vi "nc_get_NC.vi"(3 "ErrorIn":errorcluster caption="Error in", 5 "FilePath":path) -> (0 "ErrorOut":errorcluster caption="error out", 1 "NC":T1 {"vars"."NC_attrarray"."nc_type" items=["NC_NAT", "NC_BYTE", "NC_CHAR", "NC_SHORT", "NC_INT", "NC_FLOAT", "NC_DOUBLE"]; "attrs"."nc_type" items=["NC_NAT", "NC_BYTE", "NC_CHAR", "NC_SHORT", "NC_INT", "NC_FLOAT", "NC_DOUBLE"]}, 2 "refnum out":refnum<file>)   [LabVIEW 2016]
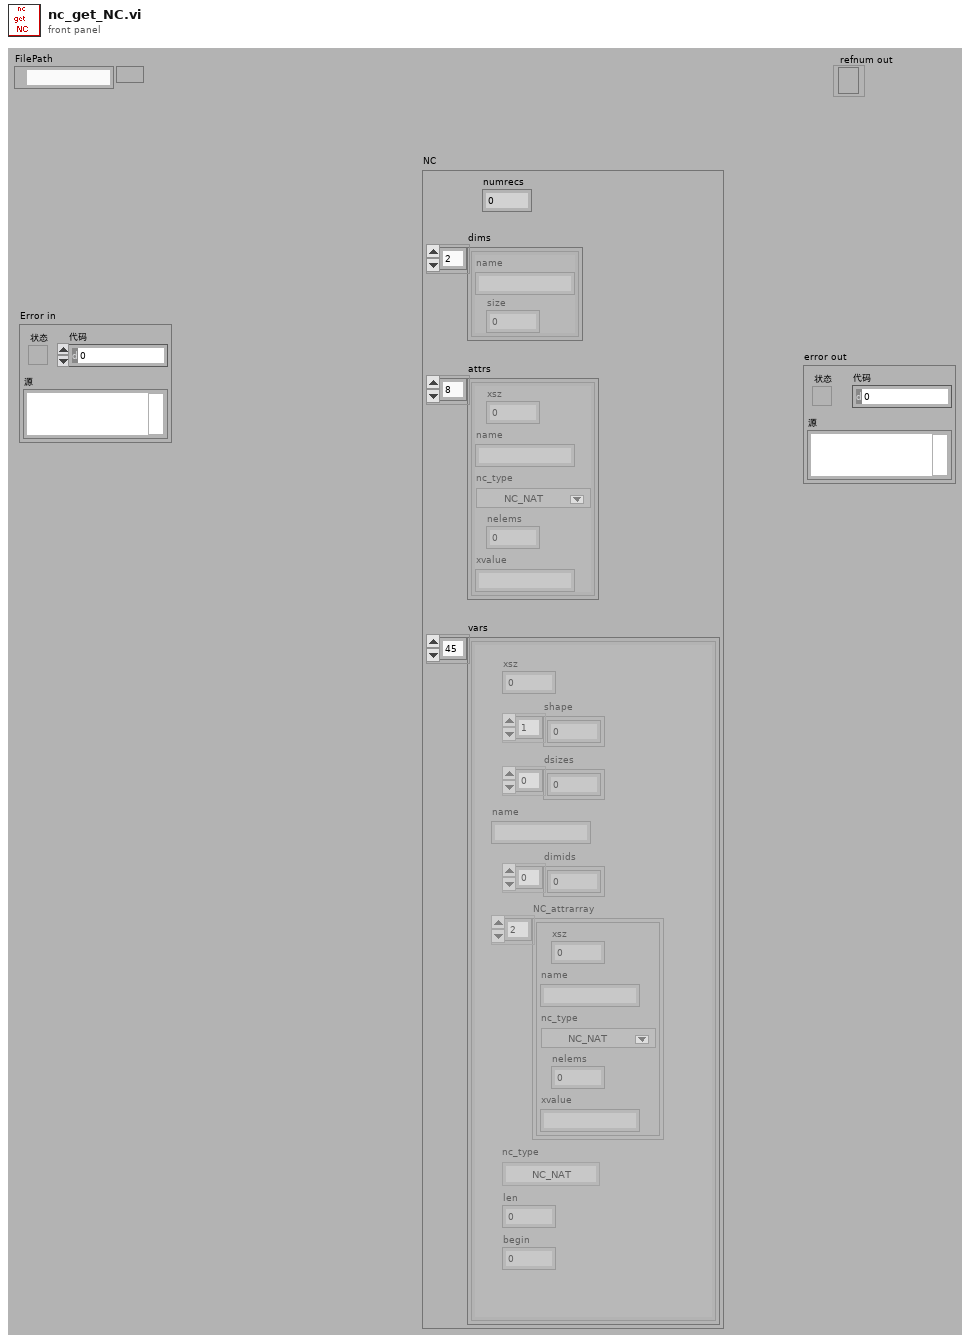
[diagram p1: front panel]
types:
  T1 = cluster{"numrecs":u64, "dims":cluster{"name":string, "size":u64}[], "attrs":cluster{"xsz":u64, "name":string, "nc_type":u16, "nelems":u64, "xvalue":string}[], "vars":cluster{"xsz":u64, "shape":u64[], "dsizes":u64[], "name":string, "dimids":u64[], "NC_attrarray":cluster{"xsz":u64, "name":string, "nc_type":u16, "nelems":u64, "xvalue":string}[], "nc_type":enum16{"NC_NAT", "NC_BYTE", "NC_CHAR", "NC_SHORT", "NC_INT", "NC_FLOAT", "NC_DOUBLE"}, "len":u64, "begin":u64}[]}
  T2 = enum16{"open", "replace", "create", "open or create", "replace or create", "replace or create with confirmation"}
  T3 = cluster{"xsz":u64, "name":string, "nc_type":u16, "nelems":u64, "xvalue":string}[]
  T4 = cluster{"xsz":u64, "shape":u64[], "dsizes":u64[], "name":string, "dimids":u64[], "NC_attrarray":cluster{"xsz":u64, "name":string, "nc_type":u16, "nelems":u64, "xvalue":string}[], "nc_type":enum16{"NC_NAT", "NC_BYTE", "NC_CHAR", "NC_SHORT", "NC_INT", "NC_FLOAT", "NC_DOUBLE"}, "len":u64, "begin":u64}[]
  T5 = cluster{"int32":i32, "NC_dimarray":cluster{"name":string, "size":u64}[], "NC_attrarray":cluster{"xsz":u64, "name":string, "nc_type":u16, "nelems":u64, "xvalue":string}[], "NC_vararray":cluster{"xsz":u64, "shape":u64[], "dsizes":u64[], "name":string, "dimids":u64[], "NC_attrarray":cluster{"xsz":u64, "name":string, "nc_type":u16, "nelems":u64, "xvalue":string}[], "nc_type":enum16{"NC_NAT", "NC_BYTE", "NC_CHAR", "NC_SHORT", "NC_INT", "NC_FLOAT", "NC_DOUBLE"}, "len":u64, "begin":u64}[]}
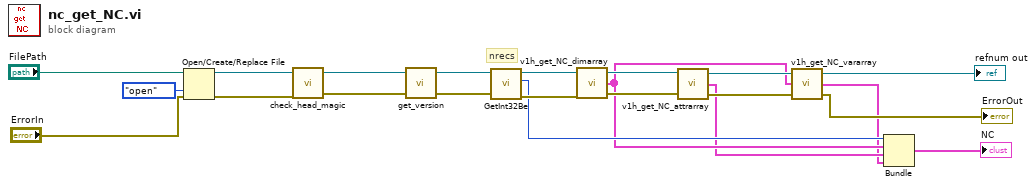
[diagram p0: block diagram]
diagram:
  # "nrecs"
  n1 = Open/Create/Replace File(file path (use dialog)="FilePath", error in="ErrorIn", operation (0:open)=T2."open" ("操作(0:open)")) -> (refnum out=w14:refnum<file>, error out=w20:errorcluster)  [unwired: 3 in, 1 out]
  n2 = call "check_head_magic.vi"("error in"=w20, "refnum in"=w14) -> ("error out"=w19:errorcluster, "refnum out"=w15:refnum<file>)  [unwired: 2 out]
  n3 = call "get_version.vi"("error in"=w19, "refnum in"=w15) -> ("error out"=w18:errorcluster, "refnum out"=w9:refnum<file>)  [unwired: 2 out]
  n4 = call "GetInt32Be.vi"("error in (no error)"=w18, "refnum in"=w9) -> ("error out"=w11:errorcluster, "int32"=w4:i32, "refnum out"=w10:refnum<file>)  [unwired: 3 out]
  n5 = call "v1h_get_NC_dimarray.vi"("error out"=w11, "refnum in"=w10) -> ("error out"=w16:errorcluster, "NC_dimarray"=w3:cluster{"name":string, "size":u64}[], "refnum out"=w12:refnum<file>)  [unwired: 1 out]
  n6 = call "v1h_get_NC_attrarray.vi"("error in (no error)"=w16, "refnum in"=w12) -> ("error out"=w17:errorcluster, "NC_attrarray"=w2:T3, "refnum out"=w13:refnum<file>)  [unwired: 1 in]
  n7 = call "v1h_get_NC_vararray.vi"("error in (no error)"=w17, "NC_dimarray"=w3, "refnum in"=w13) -> ("error out"=→"ErrorOut":errorcluster, "NC_vararray"=w1:T4, "refnum out"=→"refnum out":refnum<file>)
  n8 = Bundle("int32"=w4, "NC_dimarray"=w3, "NC_attrarray"=w2, "NC_vararray"=w1) -> (→"NC":T5)  [unwired: 1 out]
